vi "SampleRelativeMoveLoop.vi"(2 "Relative Steps":i32, 3 "Motor Number":i32=1) -> (0 "error out":errorcluster)   [LabVIEW 2016]
panel:
  out "End position":i32
  out "Initial position":i32
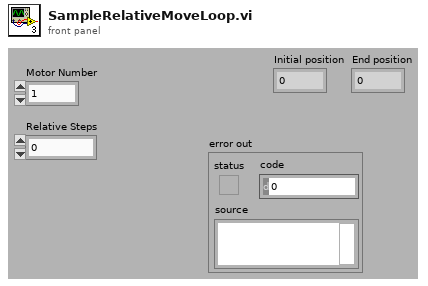
[diagram p1: front panel]
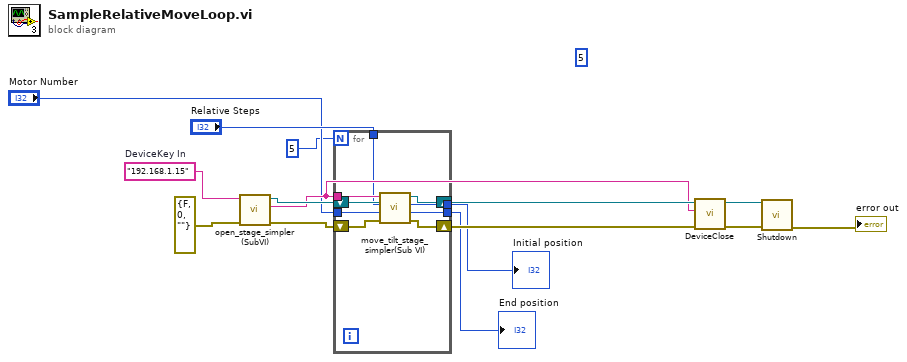
[diagram p0: block diagram]
diagram:
  (unwired) 5
  w15 = "192.168.1.15"  # DeviceKey In
  n1 = call "open_stage_simpler (SubVI).vi"("error in (no error)"=errorcluster {"status"=FALSE, "code"=0, "source"=""}, "IP address"=w15) -> ("error out"=w12:errorcluster, "deviceKey"=w7:string, "reference"=w13:refnum<k24>)  [unwired: 7 in]
  n2 = for {
    N: 5 -> [_]
    tunnel: w7 -> [w20]
    tunnel: "Relative Steps" -> [w19]
    tunnel: "Motor Number" -> [w18]
    tunnel: [w17] -> w4
    tunnel: [w16] -> w3
    shift-right: [w22] -> w11
    shift-left: w13 -> [w24]
    shift-right: [w21] -> w10
    shift-left: w12 -> [w23]
    n3 = call "move_tilt_stage_simpler(Sub VI).vi"(".NET Refnum in"=w24, "error in (no error)"=w23, "motor"=w18, "relativeSteps"=w19, "deviceKey"=w20) -> ("error out"=w21:errorcluster, "End position"=w16:i32, "Initial position"=w17:i32, ".NET Refnum out"=w22:refnum<k24>)
  }
  "Initial position" <- w4
  "End position" <- w3
  n4 = call "DeviceClose.vi"("error in (no error)"=w10, "DeviceKey In"=w7, "CmdLib In"=w11) -> ("error out"=w8:errorcluster, "CmdLib Out"=w9:refnum<k24>)  [unwired: 2 in, 1 out]
  n5 = call "Shutdown.vi"("error in (no error)"=w8, "CmdLib In"=w9) -> ("error out"=→"error out":errorcluster)  [unwired: 4 in, 1 out]
